vi "updateSettings.vi"(8 "error in (no error)":errorcluster, 9 "ID":u32, 10 "Serial Number":string, 11 "Sonometro in":refnum<class "Sonometro.lvclass">) -> (0 "error out":errorcluster, 3 "Sonometro out":refnum<class "Sonometro.lvclass">)   [LabVIEW 2019, in "Sonometro.lvclass"]
uses:
  Sonometro.lvclass
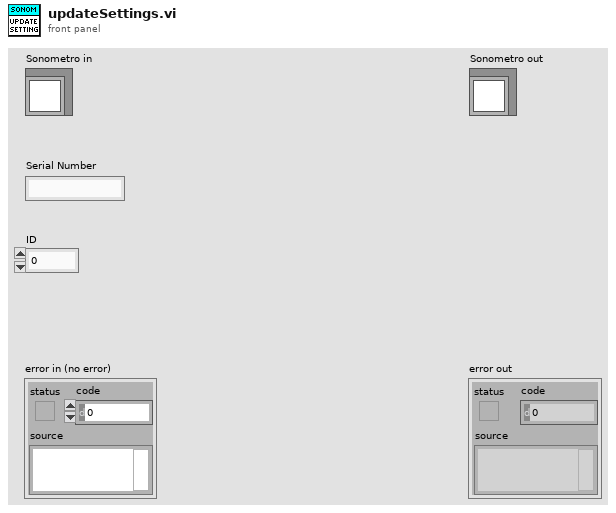
[diagram p1: front panel]
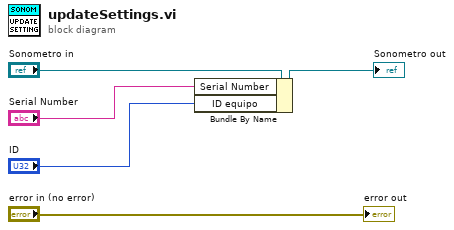
[diagram p0: block diagram]
diagram:
  n1 = Bundle By Name(cluster="Sonometro in", "Serial Number"="Serial Number", "ID equipo"="ID") -> (→"Sonometro out":refnum<class "Sonometro.lvclass">)
  "error out" <- "error in (no error)"
